vi "Record Path.vi"(9 "Record Path":bool) -> ()   [LabVIEW 2020]
uses:
  Framework/Robot Global Data.vi
  <vilib>/Analysis/Matrix/Numeric/Conversions/Matrix To Array - RM.vi
  <vilib>/Utility/file.llb/Write Delimited Spreadsheet (DBL).vi
  <vilib>/Analysis/Matrix/NI_Matrix.lvlib
panel:
  out "Path increases":dbl
  out "error out":errorcluster
  out "path":path
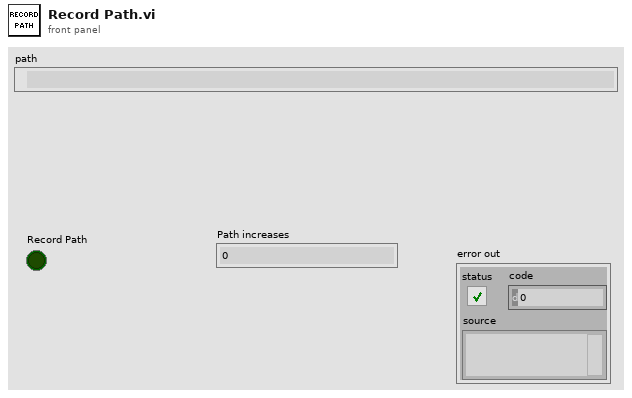
[diagram p1: front panel]
types:
  T1 = typedef "NI_Matrix.lvlib/RealMatrix.ctl" = dbl[][]
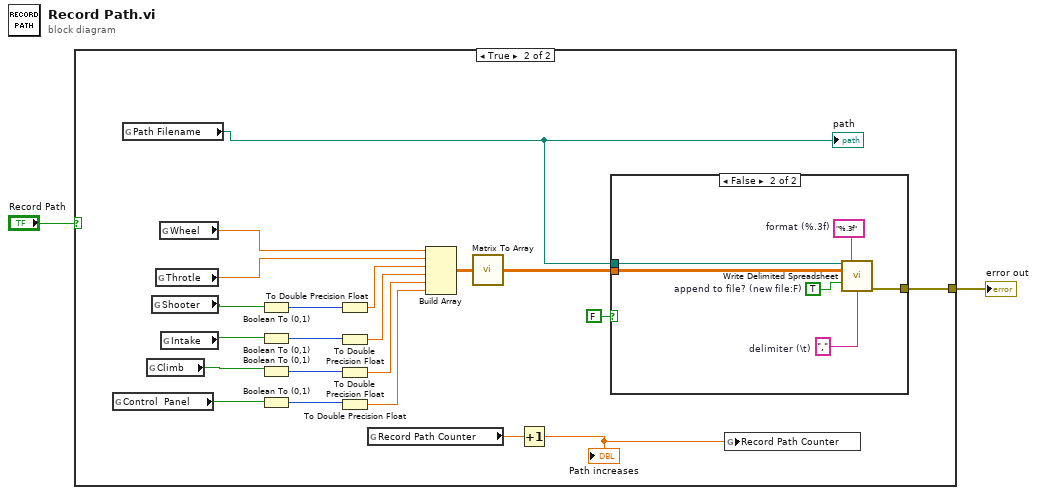
[diagram p0: block diagram]
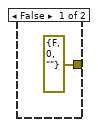
[diagram p2: hidden frame]
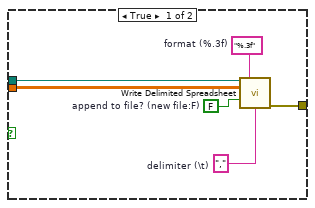
[diagram p3: hidden frame]
diagram:
  n1 = case shown="True" "Record Path" {
    tunnel: [errorcluster {"status"=FALSE, "code"=0, "source"=""} ("error out") w8] -> w1
    frame False {
    }
    frame True {
      n2 = global read "Robot Global Data.vi" "Control  Panel"() -> (w9:bool)
      n3 = global read "Robot Global Data.vi" "Path Filename"() -> (w5:path)
      "path" <- w5
      n4 = global read "Robot Global Data.vi" "Climb"() -> (w10:bool)
      n5 = global read "Robot Global Data.vi" "Shooter"() -> (w12:bool)
      n6 = global read "Robot Global Data.vi" "Throtle"() -> (w13:dbl)
      n7 = global read "Robot Global Data.vi" "Wheel"() -> (w14:dbl)
      n8 = global read "Robot Global Data.vi" "Intake"() -> (w11:bool)
      n9 = Boolean To (0,1)(Boolean=w12) -> (0, 1=w22:i16)
      n10 = Boolean To (0,1)(Boolean=w11) -> (0, 1=w21:i16)
      n11 = Boolean To (0,1)(Boolean=w10) -> (0, 1=w20:i16)
      n12 = Boolean To (0,1)(Boolean=w9) -> (0, 1=w19:i16)
      n13 = To Double Precision Float(number=w22) -> (double precision float=w18:dbl)
      n14 = To Double Precision Float(number=w21) -> (double precision float=w17:dbl)
      n15 = To Double Precision Float(number=w20) -> (double precision float=w16:dbl)
      n16 = To Double Precision Float(number=w19) -> (double precision float=w15:dbl)
      n17 = global read "Robot Global Data.vi" "Record Path Counter"() -> (w7:dbl)
      n18 = Build Array(w14, w13, w18, w17, w16, w15) -> (w24:T1)
      n19 = call-poly <vilib>:"Matrix To Array.vi"("Real Matrix"=w24) -> ("Real 2D Array"=w23:dbl[][])
      n20 = Increment(x=w7) -> (x+1=w6:dbl)
      "Path increases" <- w6
      n21 = case shown="False" FALSE {
        tunnel: w23 -> [w30 w36]
        tunnel: w5 -> [w26 w32]
        tunnel: [w25 w31] -> w8
        frame True {
          w28 = FALSE  # append to file? (new file:F)
          w29 = "%.3f"  # format (%.3f)
          w27 = ","  # delimiter (\t)
          n22 = call-poly <vilib>:"Write Delimited Spreadsheet.vi"("file path (dialog if empty)"=w26, "format (%.3f)"=w29, "2D data"=w30, "append to file? (new file:F)"=w28, "delimiter (\\t)"=w27) -> ("error out"=w25:errorcluster)  [unwired: 9 in, 1 out]
        }
        frame False {
          w34 = TRUE  # append to file? (new file:F)
          w35 = "%.3f"  # format (%.3f)
          w33 = ","  # delimiter (\t)
          n23 = call-poly <vilib>:"Write Delimited Spreadsheet.vi"("file path (dialog if empty)"=w32, "format (%.3f)"=w35, "2D data"=w36, "append to file? (new file:F)"=w34, "delimiter (\\t)"=w33) -> ("error out"=w31:errorcluster)  [unwired: 9 in, 1 out]
        }
      }
      n24 = global write "Robot Global Data.vi" "Record Path Counter"(w6) -> ()
    }
  }
  "error out" <- w1
